vi "debug_trace.vi"() -> ()   [LabVIEW 2017]
doc: "Illustrates how to register for debug trace events."
uses:
  libssh2/libssh2_session_handshake_tcp.vi
  libssh2/libssh2_init_default.vi
  libssh2/libssh2_session_init_ex.vi
  <vilib>/Utility/tcp.llb/TCP Get Raw Net Object.vi
  libssh2/libssh2_session_handshake_socket.vi
  libssh2/libssh2_userauth_password_ex.vi
  libssh2/libssh2_channel_open_ex.vi
  libssh2/libssh2_channel_process_startup.vi
  libssh2/libssh2_channel_read_ex.vi
  libssh2/libssh2.lvlib
panel:
  in  "bitmask":i32(ring)=128 items=["LIBSSH2_TRACE_TRANS"=2, "LIBSSH2_TRACE_KEX"=4, "LIBSSH2_TRACE_AUTH"=8, "LIBSSH2_TRACE_CONN"=16, "LIBSSH2_TRACE_SCP"=32, "LIBSSH2_TRACE_SFTP"=64, "LIBSSH2_TRACE_ERROR"=128, "LIBSSH2_TRACE_PUBLICKEY"=256, "LIBSSH2_TRACE_SOCKET"=512]
  out "trace output":string
  out "Output":string
  out "exitsignal":string
  out "exit status":i32
  in  "command":string="ping localhost -c 1"
  in  "password":string
  in  "username":string
  out "error out":errorcluster
  in  "hostname":string="localhost"
  # "Important\nThis only works when libssh2 is configured with \"ENABLE_DEBUG_LOGGING=ON\" on a debug build."
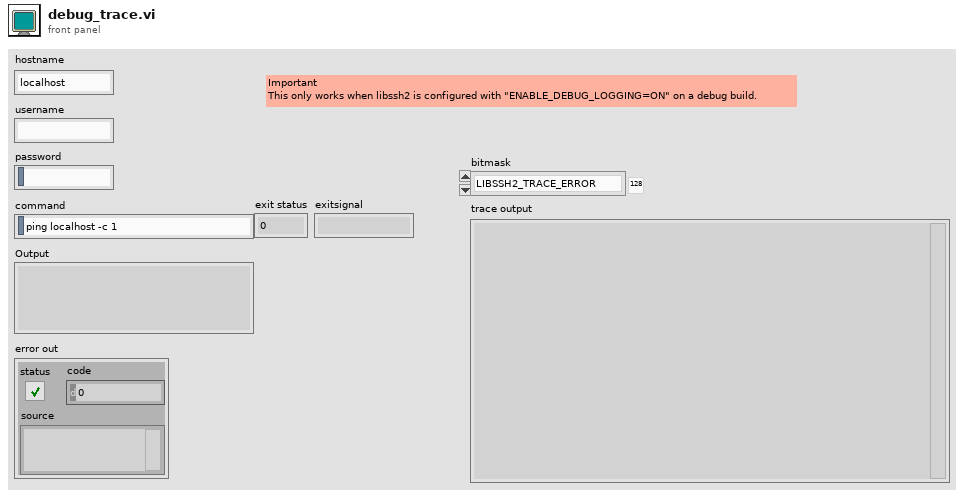
[diagram p1: front panel]
types:
  T1 = typedef "libssh2.lvlib/Session Refnum.ctl" = refnum<k1>
  T2 = typedef "libssh2.lvlib/Channel Refnum.ctl" = refnum<k1>
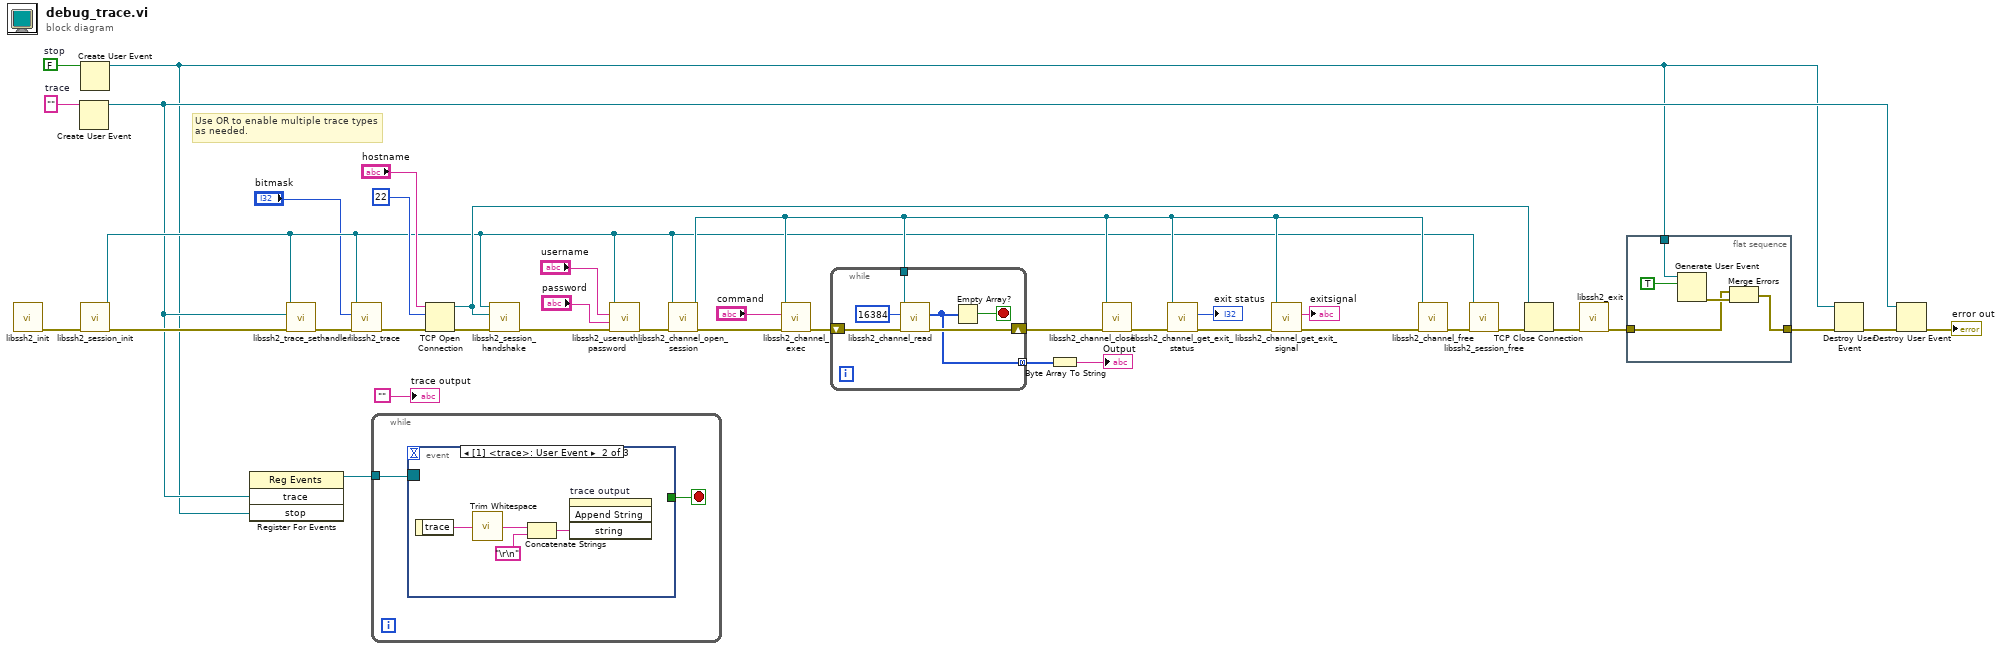
[diagram p0: block diagram]
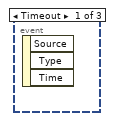
[diagram p2: hidden frame]
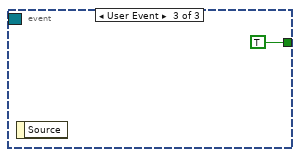
[diagram p3: hidden frame]
diagram:
  w8 = FALSE  # stop
  w11 = ""  # trace
  # "Use OR to enable multiple trace types\nas needed."
  n1 = call-poly "libssh2_init.vi"() -> ("error out"=w39:errorcluster)  [unwired: 11 in]
  n2 = Create User Event(user event datatype=w11) -> (user event=w4:refnum<user-event>)  [unwired: 1 in, 1 out]
  n3 = Create User Event(user event datatype=w8) -> (user event=w3:refnum<user-event>)  [unwired: 1 in, 1 out]
  n4 = call "libssh2_session_init.vi"("error in (no error)"=w39) -> ("error out"=w38:errorcluster, "session"=w10:T1)  [unwired: 9 in]
  n5 = register-events(w4, w3) -> (reference out=w9:refnum<event-registration>)  [unwired: 2 in, 1 out]
  n6 = call "libssh2_trace_sethandler.vi"("error in (no error)"=w38, "context"=w4, "session"=w10) -> ("error out"=w12:errorcluster)  [unwired: 8 in]
  n7 = call "libssh2_trace.vi"("error in (no error)"=w12, "bitmask"="bitmask", "session"=w10) -> ("error out"=w13:errorcluster)  [unwired: 8 in]
  n8 = while {
    tunnel: w9 -> [w41]
    stop <- w40 stop-if-true
    n9 = event shown="[1] <trace>: User Event" {
      selector: w41 -> [_ _ _]
      dyn-events: _ -> [_ _ _]
      timeout: _ -> [_ _ _]
      tunnel: [_ _ TRUE] -> w40
      event Timeout {
        n10 = event-data() -> ()  [unwired: 1 in, 3 out]
      }
      event User Event {
        n11 = event-data() -> ("trace"=w44:string)  [unwired: 1 in]
        n12 = call <vilib>:"Trim Whitespace.vi"("string"=w44) -> ("trimmed string"=w42:string)  [unwired: 1 in]
        n13 = Concatenate Strings(w42, "\r\n") -> (w43:string)
        n14 = invoke on="trace output" class="Str" method="Append String"("string"=w43) -> ()  [unwired: 3 in, 4 out]
      }
      event User Event {
        n15 = event-data() -> ()  [unwired: 1 in, 1 out]
      }
    }
  }
  n16 = TCP Open Connection(address="hostname", remote port or service name=u16 22, error in (no error)=w13) -> (connection ID=w15:refnum<k5>, error out=w16:errorcluster)  [unwired: 2 in]
  n17 = call-poly "libssh2_session_handshake.vi"("error in (no error)"=w16, "tcp connection"=w15, "session"=w10) -> ("error out"=w14:errorcluster)  [unwired: 8 in]
  n18 = call "libssh2_userauth_password.vi"("error in (no error)"=w14, "password"="password", "username"="username", "session"=w10) -> ("error out"=w33:errorcluster)  [unwired: 7 in]
  n19 = call "libssh2_channel_open_session.vi"("error in (no error)"=w33, "session"=w10) -> ("error out"=w30:errorcluster, "channel"=w22:T2)  [unwired: 8 in]
  n20 = call "libssh2_channel_exec.vi"("error in (no error)"=w30, "command"="command", "channel"=w22) -> ("error out"=w29:errorcluster)  [unwired: 8 in]
  n21 = while {
    tunnel: w22 -> [w49]
    tunnel: [w47] -> w20 mode=concatenating
    shift-right: [w51] -> w27
    shift-left: w29 -> [w52]
    stop <- w48 stop-if-true
    n22 = call "libssh2_channel_read.vi"("error in (no error)"=w52, "buffer length"=16384 ("buflen"), "channel"=w49) -> ("error out"=w51:errorcluster, "buffer"=w47:u8[])  [unwired: 7 in]
    n23 = Empty Array?(array=w47) -> (empty?=w48:bool)
  }
  n24 = Byte Array To String(unsigned byte array=w20) -> (string=→"Output":string)
  n25 = call "libssh2_channel_close.vi"("error in (no error)"=w27, "channel"=w22) -> ("error out"=w26:errorcluster)  [unwired: 9 in]
  n26 = call "libssh2_channel_get_exit_status.vi"("error in (no error)"=w26, "channel"=w22) -> ("error out"=w25:errorcluster, "exit status"=→"exit status":i32)  [unwired: 8 in]
  n27 = call "libssh2_channel_get_exit_signal.vi"("error in (no error)"=w25, "channel"=w22) -> ("error out"=w24:errorcluster, "exitsignal"=→"exitsignal":string)  [unwired: 6 in, 2 out]
  n28 = call "libssh2_channel_free.vi"("error in (no error)"=w24, "channel"=w22) -> ("error out"=w23:errorcluster)  [unwired: 9 in]
  n29 = call "libssh2_session_free.vi"("error in (no error)"=w23, "session"=w10) -> ("error out"=w37:errorcluster)  [unwired: 9 in]
  n30 = TCP Close Connection(connection ID=w15, error in (no error)=w37) -> (error out=w18:errorcluster)  [unwired: 1 in, 1 out]
  n31 = call "libssh2_exit.vi"("error in (no error)"=w18) -> ("error out"=w36:errorcluster)  [unwired: 10 in]
  n32 = flat-sequence {
    tunnel: w36 -> [w54]
    tunnel: [w55] -> w7
    tunnel: w3 -> [w56]
    frame #0 {
      n33 = Generate User Event(user event=w56, event data cluster=TRUE ("event data")) -> (error out=w57:errorcluster)  [unwired: 2 in, 1 out]
      n34 = Merge Errors(w54, w57) -> (w55:errorcluster)
    }
  }
  n35 = Destroy User Event(user event=w3, error in=w7) -> (error out=w6:errorcluster)
  n36 = Destroy User Event(user event=w4, error in=w6) -> (error out=→"error out":errorcluster)
  "trace output" <- ""
